vi "AB_RW_Convert_Path_Tags.vi"(7 "buildObject":T2, 8 "error in (no error)":errorcluster, 10 "action":T1, 11 "Path in":path) -> (0 "error out":errorcluster, 3 "Path out":path)   [LabVIEW 2020]
uses:
  <resource>/Framework/Providers/API/ItemRef.ctl
  <vilib>/AppBuilder/RW_Project/AB_RW_Project_PropBag_Action.ctl
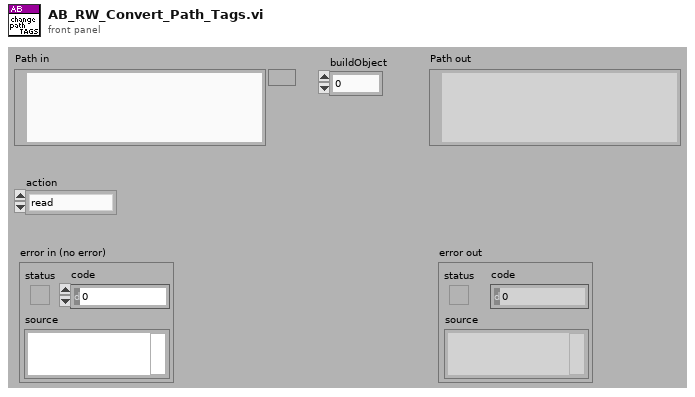
[diagram p1: front panel]
types:
  T1 = typedef "AB_RW_Project_PropBag_Action.ctl" = enum16{"read", "write", "clear", "readPrevious", "writePrevious", "clearPrevious"}
  T2 = typedef "ItemRef.ctl" = u64
  T3 = cluster{"filename without extension":string, "new label":string}
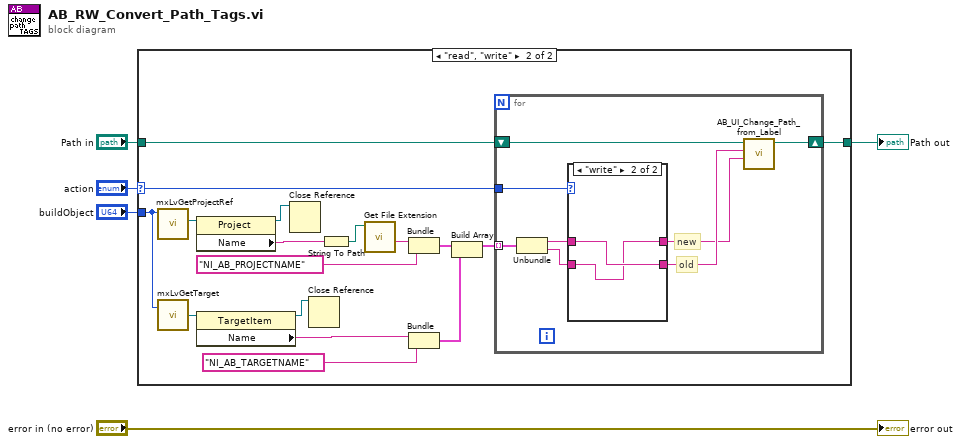
[diagram p0: block diagram]
diagram:
  n1 = case shown="\"read\", \"write\"" "action" {
    selector: "action" -> [_ w21]
    tunnel: "buildObject" -> [_ w12]
    tunnel: "Path in" -> [w6 w19]
    tunnel: [w6 w20] -> w2
    frame Default {
    }
    frame "read", "write" {
      n2 = call <resource>:"mxLvGetProjectRef.vi"("Item"=w12) -> ("Project Refnum"=w23:refnum<vi>)  [unwired: 1 in, 9 out]
      n3 = call <resource>:"mxLvGetTarget.vi"("Item"=w12) -> ("Target"=w11:refnum<vi>)  [unwired: 1 in, 2 out]
      n4 = property class="Project"(reference=w23) -> (reference out=w22:refnum<vi>, "Name"=w17:string)  [unwired: 1 in, 1 out]
      n5 = property class="TargetItem"(reference=w11) -> (reference out=w7:refnum<vi>, "Name"=w10:string)  [unwired: 1 in, 1 out]
      n6 = Close Reference(reference=w22) -> ()  [unwired: 1 in, 1 out]
      n7 = Close Reference(reference=w7) -> ()  [unwired: 1 in, 1 out]
      n8 = String To Path(string=w17) -> (path=w18:path)
      n9 = call <vilib>:"Get File Extension.vi"("file"=w18) -> ("filename without extension"=w16:string)  [unwired: 1 in, 9 out]
      n10 = Bundle("filename without extension"=w16, "new label"="NI_AB_PROJECTNAME") -> (w15:T3)  [unwired: 1 out]
      n11 = Bundle("Name"=w10, "new label"="NI_AB_TARGETNAME") -> (w8:cluster{"Name":string, "new label":string})  [unwired: 1 out]
      n12 = Build Array(w15, w8) -> (w13:cluster{"Name":string, "new label":string}[])
      n13 = for {
        tunnel: w21 -> [w31]
        shift-right: [w30] -> w20
        shift-left: w19 -> [w27]
        tunnel: w13 -> [w26] mode=indexing
        # "new"
        # "old"
        n14 = Unbundle(w26) -> ("Name"=w25:string, "new label"=w24:string)
        n15 = case shown="\"write\"" w31 {
          tunnel: w25 -> [w32 w35]
          tunnel: w24 -> [w33 w34]
          tunnel: [w33 w35] -> w29
          tunnel: [w32 w34] -> w28
          frame "read", Default {
          }
          frame "write" {
          }
        }
        n16 = call <resource>:"AB_UI_Change_Path_from_Label.vi"("new label"=w28, "old label"=w29, "Path in"=w27) -> ("Path out"=w30:path)  [unwired: 1 in, 7 out]
      }
    }
  }
  "Path out" <- w2
  "error out" <- "error in (no error)"
